vi "DIALOG_Cluster Item Selection.vi"(7 "Action":T15=enum."Bundler Insert", 8 "Error In":errorcluster, 9 "User VI Ref":refnum<vi>, 10 "Affected Items":T13, 11 "Display Items":T14[](array[typedef])) -> (0 "Error Out":errorcluster, 2 "Action Choice Out":enum32{"Choice 1", "Choice 2"}(radio), 3 "Selected Items (tags)":string[](array[string]))   [LabVIEW 2023]
doc: "Dialog to select items from the input cluster ref. \n\nFilter narrows list of items.\nDown key puts focus on tree and selects first item.\nUp and Down keps navigate tree.\nMultiple items can be selected.\n\nIn case of action \"Delete\" (\"Remove elements(s)...\" selected), list will show all elements currently displayed, else it will show all elements availabel to undle or unbundle.\n\nOutput is a list of the selected item tags.\n\nSelected element is the item clicked in a bundler node, displayed ot help user remember where an insert will happen."
uses:
  controls/action enum.ctl
  cluster/Cluster Element Description.ctl
  top/BundleMagic.ctl
  eero compliance/eero-Compliance-5m-Chamber/Code/Config/Equipment/Motion Control Max Speed.ctl
  eero compliance/eero-Compliance-5m-Chamber/Code/Scan/Spurious Emissions/controls/RSE_SA Settings Cluster.ctl
  eero compliance/eero-Compliance-5m-Chamber/Code/Equipment/rhode_schwartz/Controls/Trace Types Enum.ctl
  eero compliance/eero-Compliance-5m-Chamber/Code/Sequence/Controls/Prescan Steps Cluster.ctl
  eero compliance/eero-Compliance-5m-Chamber/Code/Controls/Start Stop Step Cluster.ctl
  eero compliance/eero-Compliance-5m-Chamber/Code/Sequence/Controls/Polarization Radio Buttons.ctl
  eero compliance/eero-Compliance-5m-Chamber/Code/Sequence/Controls/Sequence Motion Control Order Enum.ctl
  eero compliance/eero-Compliance-5m-Chamber/Code/Sequence/Controls/RSE_EUT Settings.ctl
  eero compliance/eero-Compliance-5m-Chamber/Code/Equipment/eero device driver/controls/eero model.ctl
  eero compliance/eero-Compliance-5m-Chamber/Code/Sequence/Controls/EUT Command Cluster.ctl
  eero compliance/eero-Compliance-5m-Chamber/Code/Sequence/Controls/Zoom Scan Steps Cluster.ctl
  LabVIEW-common/Controls/Get-Set Enum.ctl
panel:
  in  "Filter":string
  in  "Tree":string[](tree)
  in  "Select Unwired":bool
  out "Selected Element String":string
  in  "Action Choice Radio Buttons":enum32{"Choice 1", "Choice 2"}(radio)
  in  "Done":bool
  in  "Cluster":T12={"Cont?"=TRUE, "Config File Path"=path "", "Max Speeds"={"Mast V (cm/s)"=0.0, "Mast A (cm/s^2)"=0.0, "Turntable V (deg/s)"=0.0, "Turntable A (deg/s^2)"=0.0, "Polarization (s)"=0.0}, "Scan Speeds"={"Mast V (cm/s)"=0.0, "Mast A (cm/s^2)"=0.0, "Turntable V (deg/s)"=0.0, "Turntable A (deg/s^2)"=0.0, "Polarization (s)"=0.0}, "Sequence Order Override"=TRUE, "Sequence Timing Listbox Ref"=refnum, "Spectrum Analyzer Config"={"Start Frequency"=3000000000.0, "Stop Frequency"=18000000000.0, "Resolution BW"=1000000.0, "Video BW"=3000000.0, "Sweep Time"=1.0, "Trace 1 Detector"=1, "Trace 2 Detector"=3, "Sweep Points"=10001}, "Limit Line Enums"=[], "Calib Listbox Ref"=refnum, "Correction Paths"=[], "Seq Path"=path "", "Motion Settings"={"Mast"={"Start"=0.0, "Stop"=0.0, "Step"=0.0}, "Turntable"={"Start"=0.0, "Stop"=0.0, "Step"=0.0}, "Polarizations"={"H"=TRUE, "V"=TRUE}, "Sequence Order"=enum."Height-Pol-Angle"}, "EUT Settings"={"Model"=enum."Unico", "Command Array"=[]}, "Limit Paths"=[], "Zoom Steps"={"Mast Adjustment Range (cm)"=5.0, "Mast Step Size (cm)"=10.0, "Turntable Adjustment Range (deg)"=0.0, "Turntable Step Size (deg)"=5.0}} {"Spectrum Analyzer Config"."Trace 2 Detector" items=["", "Average", "Maximum Peak", "Minimum Peak", "RMS", "QPeak", "Cispr RMS", "Cispr Average"]; "Spectrum Analyzer Config"."Trace 1 Detector" items=["", "Average", "Maximum Peak", "Minimum Peak", "RMS", "QPeak", "Cispr RMS", "Cispr Average"]; "Spectrum Analyzer Config"."Sweep Time" format="%#_13g"; "Spectrum Analyzer Config"."Video BW" format="%#_13e"; "Spectrum Analyzer Config"."Resolution BW" format="%#_13e"; "Spectrum Analyzer Config"."Stop Frequency" format="%^.3e"; "Spectrum Analyzer Config"."Start Frequency" format="%^.3e"}
  in  "Show radio":bool
  in  "C1":T16
  # "All panes scroll to origin at runtime, so we don't have to worry about pane placements\n\nThis pane contracts at runtime and vertical splitter to left sticks to right at runtime so resizing functions happen as expected."
  # "Debug"
  # "Debug Cluster"
  # "(Use for debug if display items empty)"
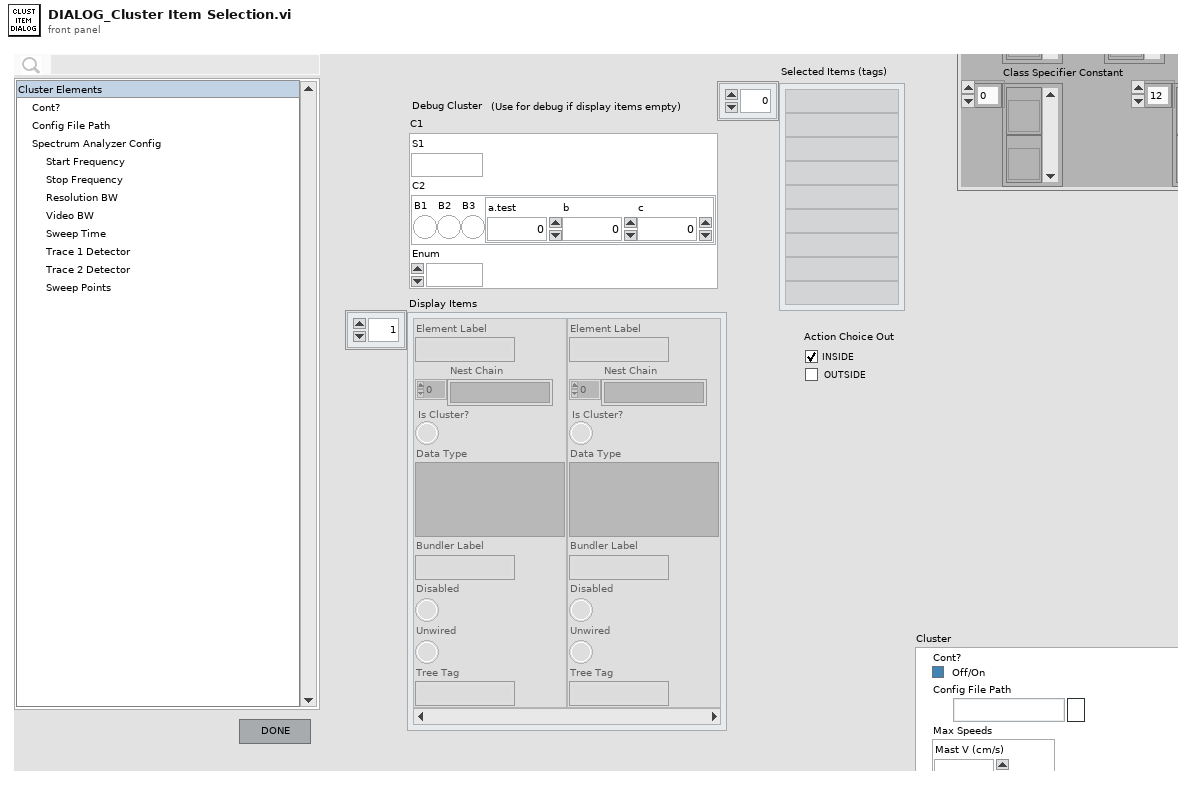
[diagram p1: front panel]
types:
  T1 = typedef "Motion Control Max Speed.ctl" = cluster{"Mast V (cm/s)":dbl, "Mast A (cm/s^2)":dbl, "Turntable V (deg/s)":dbl, "Turntable A (deg/s^2)":dbl, "Polarization (s)":dbl}
  T2 = typedef "RSE_SA Settings Cluster.ctl" = cluster{"Start Frequency":dbl, "Stop Frequency":dbl, "Resolution BW":dbl, "Video BW":dbl, "Sweep Time":dbl, "Trace 1 Detector":T3, "Trace 2 Detector":T3, "Sweep Points":u16}
  T3 = typedef "Trace Types Enum.ctl" = i32
  T4 = typedef "Prescan Steps Cluster.ctl" = cluster{"Mast":T5, "Turntable":T5, "Polarizations":T6, "Sequence Order":T7}
  T5 = typedef "Start Stop Step Cluster.ctl" = cluster{"Start":dbl, "Stop":dbl, "Step":dbl}
  T6 = typedef "Polarization Radio Buttons.ctl" = cluster{"H":bool, "V":bool}
  T7 = typedef "Sequence Motion Control Order Enum.ctl" = enum16{"Pol-Height-Angle", "Pol-Angle-Height", "Height-Angle-Pol", "Height-Pol-Angle", "Angle-Height-Pol", "Angle-Pol-Height"}
  T8 = typedef "RSE_EUT Settings.ctl" = cluster{"Model":T9, "Command Array":T10[]}
  T9 = typedef "eero model.ctl" = enum16{"Unico", "Piccino", "Cento", "Andytown-g", "Andytown-l", "Eden", "Firefly", "Trieste", "Jupiter", "Crane", "Ladro", "Merci", "Snowbird\n"}
  T10 = typedef "EUT Command Cluster.ctl" = cluster{"Command(s)":string, "Scan ID":string}
  T11 = typedef "Zoom Scan Steps Cluster.ctl" = cluster{"Mast Adjustment Range (cm)":dbl, "Mast Step Size (cm)":dbl, "Turntable Adjustment Range (deg)":dbl, "Turntable Step Size (deg)":dbl}
  T12 = cluster{"Cont?":bool, "Config File Path":path, "Max Speeds":T1, "Scan Speeds":T1, "Sequence Order Override":bool, "Sequence Timing Listbox Ref":refnum<vi>, "Spectrum Analyzer Config":T2, "Limit Line Enums":refnum<vi>[], "Calib Listbox Ref":refnum<vi>, "Correction Paths":path[], "Seq Path":path, "Motion Settings":T4, "EUT Settings":T8, "Limit Paths":path[], "Zoom Steps":T11}
  T13 = typedef "BundleMagic.ctl" = cluster{"Terminals":refnum<vi>[], "Wires":refnum<vi>[], "Named Bundler":refnum<vi>[], "Named Unbundler":refnum<vi>[], "In Place Cluster Node":refnum<vi>[], "Class Specifier Constant":refnum<vi>[], "Property Node":refnum<vi>[], "Invoke Node":refnum<vi>[], "Refnum Control":refnum<vi>[]}
  T14 = typedef "Cluster Element Description.ctl" = cluster{"Element Label":string, "Nest Chain":string[], "Is Cluster?":bool, "Data Type":variant, "Bundler Label":string, "Disabled":bool, "Unwired":bool, "Tree Tag":string}
  T15 = typedef "action enum.ctl" = enum16{"[NONE]", "Wire Bundle", "Wire Unbundle", "Terminal Unbundle", "Terminal Bundle", "Bundler Move Up", "Bundler Move Down", "Bundler Insert", "Bundler Remove", "Bundler Remove Unwired", "Bundler Rearrange", "In Place Insert", "In Place Remove", "In Place Remove Unwired", "In Place Rearrange", "Wire Properties", "Wire Method", "Terminal Properties", "Terminal Method", "Property Move Up", "Property Move Down", "Properties Insert", "Properties Remove", "Properties Remove Unwired", "Properties Rearrange", "Method Change", "Class for Constant", "Class For Control", "Class For Node", "Class Name to Clipboard"}
  T16 = cluster{"S1":string, "C2":cluster{"B1":bool, "B2":bool, "B3":bool, cluster{"a.test":dbl, "b":i32, "c":u8}}, "Enum":enum16{""}}
  T17 = typedef "Get-Set Enum.ctl" = enum16{"Get", "Set"}
  T18 = typedef "eventvkey.ctl" = enum16{"ASCII", "Enter", "Return", "Shift", "Ctrl", "Alt", "Cmd", "Opt", "Caps", "NumLock", "Clear", "Break", "Up", "Down", "Left", "Right", "Insert", "Delete", "Home", "End", "PageUp", "PageDown", "Escape", "Help", "Pause", "ScrollLock", "F1", "F2", "F3", "F4", "F5", "F6", "F7", "F8", "F9", "F10", "F11", "F12", "F13", "F14", "F15", "F16", "F17", "F18", "F19", "F20", "F21", "F22", "F23", "F24", "Play", "VolumeUp", "VolumeDown", "Mute", "Two Byte Char"}
  T19 = typedef "LVPoint32TypeDef.ctl" = cluster{"Horizontal":i32, "Vertical":i32}
  T20 = cluster{"Shift":bool, "Ctrl":bool, "Alt":bool, "Cmd":bool, "Opt":bool}
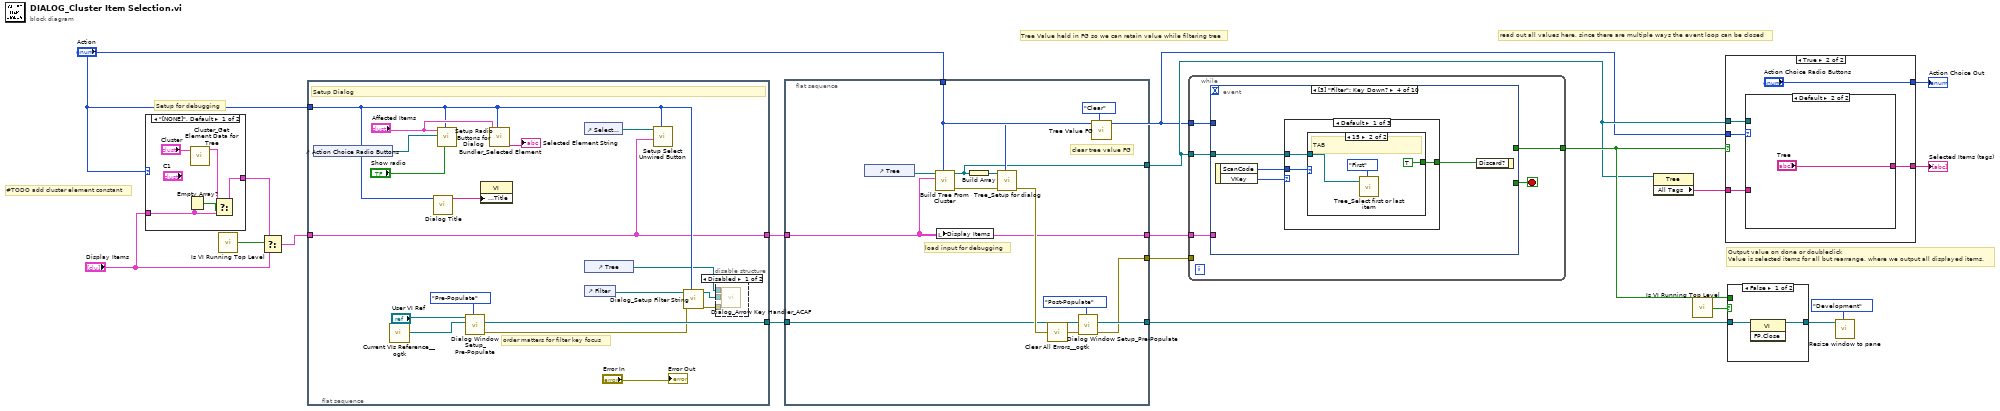
[diagram p0: block diagram]
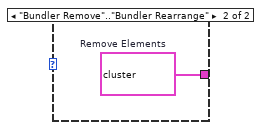
[diagram p2: hidden frame]
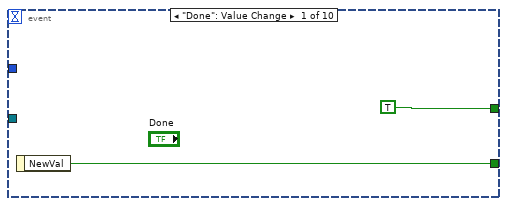
[diagram p4: hidden frame]
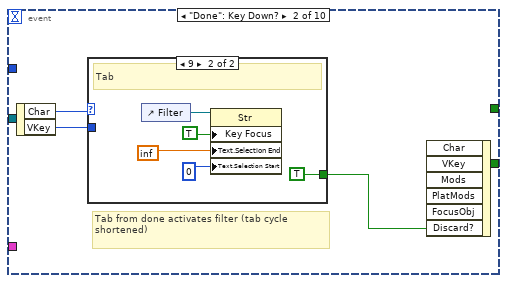
[diagram p5: hidden frame]
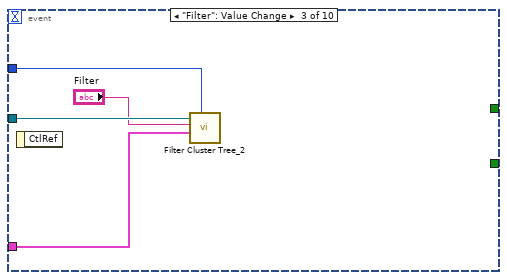
[diagram p7: hidden frame]
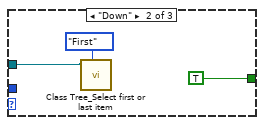
[diagram p9: hidden frame]
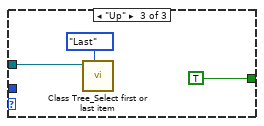
[diagram p10: hidden frame]
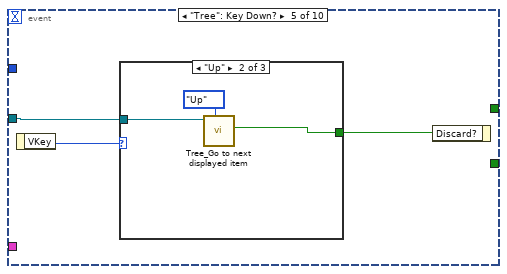
[diagram p11: hidden frame]
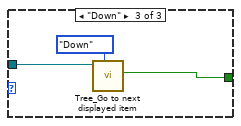
[diagram p13: hidden frame]
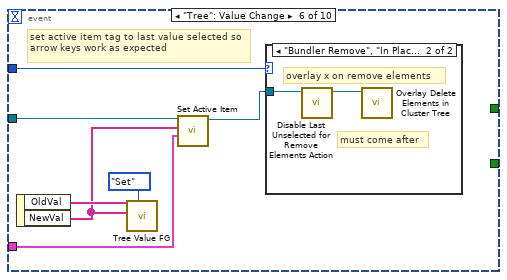
[diagram p14: hidden frame]
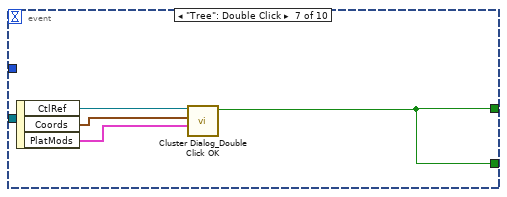
[diagram p16: hidden frame]
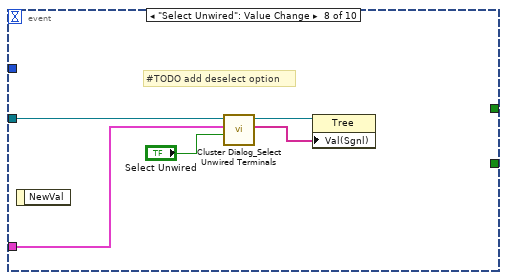
[diagram p17: hidden frame]
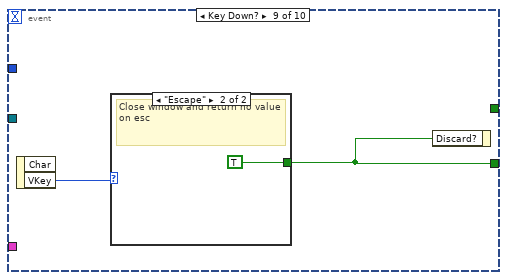
[diagram p18: hidden frame]
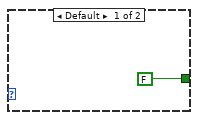
[diagram p19: hidden frame]
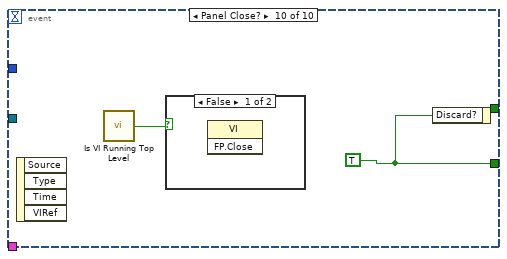
[diagram p20: hidden frame]
diagram:
  # "#TODO add cluster element constant"
  # "Setup for debugging"
  # "Tree Value held in FG so we can retain value while filtering tree"
  # "read out all values here, since there are multiple ways the event loop can be closed"
  # "Output value on done or doubleclick\nValue is selected items for all but rearrange, where we output all displayed items."
  n1 = case shown="\"[NONE]\", Default" "Action" {
    tunnel: [w21 w24] -> w4
    tunnel: "Display Items" -> [w20 _]
    frame "[NONE]", Default {
      n2 = Empty Array?(array=w20) -> (empty?=w19:bool)
      n3 = call "Cluster_Get Element Data for Tree.vi"("Data Type"="Cluster") -> ("Cluster Element Data Aray"=w22:T14[])  [unwired: 10 in]
      n4 = Select(t=w22, s=w19, f=w20) -> (s? t:f=w21:T14[])
    }
    frame "Bundler Remove".."Bundler Rearrange" {
      w24 = T14[] [{"Element Label"="N1", "Nest Chain"=[], "Is Cluster?"=FALSE, "Data Type"=variant(dbl 0.0), "Bundler Label"="N1", "Disabled"=FALSE, "Unwired"=FALSE, "Tree Tag"="0[$`~g;}N1"}, {"Element Label"="N2", "Nest Chain"=["C1"], "Is Cluster?"=TRUE, "Data Type"=variant(dbl 0.0), "Bundler Label"="C1.N2", "Disabled"=FALSE, "Unwired"=FALSE, "Tree Tag"="C1[$`~g;}C1[$`~g;}N2"}, {"Element Label"="Boolean", "Nest Chain"=["C1"], "Is Cluster?"=TRUE, "Data Type"=variant(bool FALSE), "Bundler Label"="C1.Boolean", "Disabled"=FALSE, "Unwired"=TRUE, "Tree Tag"="C2[$`~g;}C1[$`~g;}Boolean"}, {"Element Label"="C1", "Nest Chain"=[], "Is Cluster?"=FALSE, "Data Type"=variant(cluster{"N2":dbl, "Boolean":bool} {"N2"=0.0, "Boolean"=FALSE}), "Bundler Label"="C1", "Disabled"=FALSE, "Unwired"=FALSE, "Tree Tag"="3[$`~g;}C1"}, {"Element Label"="String", "Nest Chain"=[], "Is Cluster?"=FALSE, "Data Type"=variant(string ""), "Bundler Label"="String", "Disabled"=FALSE, "Unwired"=FALSE, "Tree Tag"="4[$`~g;}String"}]  # Remove Elements
    }
  }
  n5 = call "Is VI Running Top Level.vi"() -> ("Top Level?"=w5:bool)  [unwired: 5 in]
  n6 = Select(t=w4, s=w5, f="Display Items") -> (s? t:f=w3:T14[])
  n7 = flat-sequence {
    tunnel: "Action" -> [w36]
    tunnel: [w25] -> w9
    tunnel: [w32] -> w11
    tunnel: w3 -> [w25]
    frame #0 {
      # "order matters for filter key focus"
      # "Setup Dialog"
      n8 = control-ref of="Action Choice Radio Buttons"() -> (w41:refnum<vi>)
      n9 = call <userlib>:"Current VIs Reference__ogtk.vi"() -> ("Current VI's reference"=w35:refnum<vi>)  [unwired: 5 in]
      n10 = call "Dialog Title.vi"("Action"=w36) -> ("Window Title"=w39:string)  [unwired: 10 in]
      n11 = call "Setup Radio Buttons for Dialog.vi"("Show Radio"="Show radio", "Action"=w36, "Action Choice Ref"=w41, "Affected Items"="Affected Items") -> ()  [unwired: 8 in]
      n12 = call "Dialog Window Setup_Pre-Populate.vi"("Action"=enum16{"Pre-Populate", "Post-Populate"}."Pre-Populate", "Dialog VI Ref In [Parent]"=w35, "Scripted VI Ref"="User VI Ref") -> ("error out"=w29:errorcluster, "Dialog VI Ref Out"=w32:refnum<vi>)  [unwired: 7 in]
      n13 = property class="VI"("Front Panel.Title"=w39) -> ()  [unwired: 2 in, 2 out]
      n14 = call "Bundler_Selected Element.vi"("Action"=w36, "Affected Items"="Affected Items") -> ("Display String"=→"Selected Element String":string)  [unwired: 4 in, 5 out]
      n15 = control-ref of="Tree"() -> (w27:refnum<vi>)
      n16 = control-ref of="Select Unwired"() -> (w40:refnum<vi>)
      n17 = control-ref of="Filter"() -> (w30:refnum<vi>)
      n18 = call "Setup Select Unwired Button.vi"("Action"=w36, "Display Items"=w25, "Boolean in"=w40) -> ()  [unwired: 9 in]
      n19 = call "Dialog_Setup Filter String.vi"("Action"=w36, "error in"=w29, "Filter String Ref"=w30) -> ("error out"=w28:errorcluster, "Filter String Ref Out"=w26:refnum<vi>)  [unwired: 7 in]
      n20 = disable-structure shown="Disabled" {
        disable-tunnel: w28 -> [w45 _]
        disable-tunnel: w27 -> [w44 _]
        disable-tunnel: w26 -> [w43 _]
        frame Disabled {
          n21 = call "Dialog_Arrow Key Handler_ACAF.vi"("error in (no error)"=w45, "String Ref"=w43, "Tree Ref"=w44) -> ()  [unwired: 8 in, 1 out]
        }
        frame Enabled {
        }
      }
      "Error Out" <- "Error In"
    }
  }
  n22 = flat-sequence {
    tunnel: "Action" -> [w56]
    tunnel: w11 -> [w53]
    tunnel: [w52] -> w10
    tunnel: w9 -> [w46]
    tunnel: [w49] -> w8
    tunnel: [w46] -> w7
    tunnel: [w48] -> w6
    frame #0 {
      # "clear tree value FG"
      # "load input for debugging"
      n23 = control-ref of="Tree"() -> (w57:refnum<vi>)
      n24 = call "Build Tree From Cluster.vi"("Action"=w56, "Display Items"=w46, "Tree Ref"=w57) -> ("error out"=w58:errorcluster, "Tree Ref Out"=w48:refnum<vi>)  [unwired: 7 in]
      n25 = local write "Display Items"(w46) -> ()
      n26 = Build Array(w48) -> (w55:refnum<vi>[])
      n27 = call "Tree_Setup for dialog.vi"("Action"=w56, "error in"=w58, "Tree Ref"=w55) -> ("error out"=w54:errorcluster)  [unwired: 7 in, 1 out]
      n28 = call <userlib>:"Clear All Errors__ogtk.vi"("Error In"=w54) -> ("Error Out"=w50:errorcluster)  [unwired: 3 in]
      n29 = call "Dialog Window Setup_Pre-Populate.vi"("Action"=enum16{"Pre-Populate", "Post-Populate"}."Post-Populate", "error in"=w50, "Dialog VI Ref In [Parent]"=w53) -> ("error out"=w49:errorcluster, "Dialog VI Ref Out"=w52:refnum<vi>)  [unwired: 7 in]
      n30 = call "Tree Value FG.vi"("Get Set Enum"=enum16{"Get", "Set", "Clear"}."Clear") -> ()  [unwired: 10 in, 1 out]
    }
  }
  n31 = while {
    tunnel: w6 -> [w62]
    tunnel: [w61] -> w13
    tunnel: "Action" -> [w60]
    tunnel: w7 -> [w59]
    tunnel: w8 -> [_]
    stop <- w63 stop-if-true
    n32 = event shown="[3] \"Filter\": Key Down?" {
      selector: _ -> [_ _ _ _ _ _ _ _ _ _]
      dyn-events: _ -> [_ _ _ _ _ _ _ _ _ _]
      timeout: _ -> [_ _ _ _ _ _ _ _ _ _]
      tunnel: [w65 _ _ _ _ _ w115 _ w121 w126] -> w63
      tunnel: w62 -> [_ _ w77 w81 w94 w107 _ w119 _ _]
      tunnel: [TRUE _ _ _ _ _ w115 _ _ _] -> w61
      tunnel: w60 -> [_ _ w74 _ _ w109 _ _ _ _]
      tunnel: w59 -> [_ _ w75 _ _ w103 _ w120 _ _]
      event "Done": Value Change {
        n33 = event-data() -> ("NewVal"=w65:bool)  [unwired: 1 in]
      }
      event "Done": Key Down? {
        # "Tab from done activates filter (tab cycle shortened)"
        n34 = event-data() -> ("Char"=w68:i16, "VKey"=w66:T18)  [unwired: 1 in]
        n35 = case shown="9" w68 {
          tunnel: [_ TRUE ("Discard?")] -> w67
          tunnel: w66 -> [_ _]
          frame 0, Default {
          }
          frame 9 {
            # "Tab"
            n36 = control-ref of="Filter"() -> (w72:refnum<vi>)
            n37 = property class="Str"(reference=w72, "Key Focus"=TRUE, "Text.Selection End"=inf, "Text.Selection Start"=u32 0 ("Text.Selection:Start")) -> ()  [unwired: 1 in, 2 out]
          }
        }
        n38 = event-data("Discard?"=w67) -> ()  [unwired: 6 in, 1 out]
      }
      event "Filter": Value Change {
        n39 = event-data() -> ()  [unwired: 1 in, 1 out]
        n40 = call "Filter Cluster Tree_2.vi"("Action"=w74, "Display Items"=w75, "Filter Str"="Filter", "Tree Ref"=w77) -> ()  [unwired: 7 in, 1 out]
      }
      event "Filter": Key Down? {
        n41 = event-data() -> ("ScanCode"=w79:i16, "VKey"=w80:T18)  [unwired: 1 in]
        n42 = case shown="Default" w80 {
          tunnel: [w83 TRUE TRUE] -> w78
          tunnel: w81 -> [w84 w88 w92]
          tunnel: w79 -> [w82 _ _]
          frame Default {
            n43 = case shown="15" w82 {
              tunnel: w84 -> [_ w86]
              tunnel: [_ TRUE] -> w83
              frame 0, Default {
              }
              frame 15 {
                # "TAB"
                n44 = call "Tree_Select first or last item.vi"("Select Item"=enum16{"First", "Last"}."First", "Tree Ref"=w86) -> ()  [unwired: 8 in, 2 out]
              }
            }
          }
          frame "Down" {
            n45 = call "Class Tree_Select first or last item.vi"("Select Item"=enum16{"First", "Last"}."First", "Tree Ref"=w88) -> ()  [unwired: 9 in, 1 out]
          }
          frame "Up" {
            n46 = call "Class Tree_Select first or last item.vi"("Select Item"=enum16{"First", "Last"}."Last", "Tree Ref"=w92) -> ()  [unwired: 9 in, 1 out]
          }
        }
        n47 = event-data("Discard?"=w78) -> ()  [unwired: 1 in, 1 out]
      }
      event "Tree": Key Down? {
        n48 = event-data() -> ("VKey"=w96:T18)  [unwired: 1 in]
        n49 = case shown="\"Up\"" w96 {
          tunnel: [_ w97 w100] -> w95
          tunnel: w94 -> [_ w98 w101]
          frame Default {
          }
          frame "Up" {
            n50 = call "Tree_Go to next displayed item.vi"("Direction"=enum16{"Down", "Up"}."Up", "Tree ref"=w98) -> ("discard"=w97:bool)  [unwired: 7 in, 2 out]
          }
          frame "Down" {
            n51 = call "Tree_Go to next displayed item.vi"("Direction"=enum16{"Down", "Up"}."Down", "Tree ref"=w101) -> ("discard"=w100:bool)  [unwired: 7 in, 2 out]
          }
        }
        n52 = event-data("Discard?"=w95) -> ()  [unwired: 1 in, 1 out]
      }
      event "Tree": Value Change {
        # "set active item tag to last value selected so arrow keys work as expected"
        n53 = event-data() -> ("OldVal"=w106:string[], "NewVal"=w104:string[])  [unwired: 1 in]
        n54 = call "Tree Value FG.vi"("Get Set Enum"=Get-Set_Enum."Set", "NewVal"=w104, "Old Val"=w106) -> ()  [unwired: 8 in, 1 out]
        n55 = call "Set Active Item.vi"("Display Items"=w103, "NewVal"=w104, "TreeControl in"=w107) -> ("TreeControl out"=w108:refnum<vi>)  [unwired: 8 in]
        n56 = case shown="\"Bundler Remove\", \"In Place Remove\"" w109 {
          tunnel: w108 -> [_ w111]
          frame "[NONE]", Default {
          }
          frame "Bundler Remove", "In Place Remove" {
            # "overlay x on remove elements"
            # "must come after"
            n57 = call "Disable Last Unselected for Remove Elements Action.vi"("Tree Ref"=w111) -> ("Tree Ref Out"=w110:refnum<vi>)  [unwired: 8 in, 2 out]
            n58 = call "Overlay Delete Elements in Cluster Tree.vi"("Tree Ref"=w110) -> ()  [unwired: 10 in, 1 out]
          }
        }
      }
      event "Tree": Double Click {
        # "Double click to select and end entry"
        n59 = event-data() -> ("CtlRef"=w114:refnum<vi>, "Coords"=w113:T19, "PlatMods"=w112:T20)  [unwired: 1 in]
        n60 = call "Cluster Dialog_Double Click OK.vi"("PlatMods"=w112, "Coords"=w113, "TreeControl in"=w114) -> ("Valid Item Double Clicked"=w115:bool)  [unwired: 8 in]
      }
      event "Select Unwired": Value Change {
        # "#TODO add deselect option"
        n61 = event-data() -> ()  [unwired: 1 in, 1 out]
        n62 = call "Cluster Dialog_Select Unwired Terminals.vi"("Select Unwired"="Select Unwired", "Display Items"=w120, "Tree Ref"=w119) -> ("Selected items"=w116:string[], "Tree Ref Out"=w117:refnum<vi>)  [unwired: 7 in]
        n63 = property class="Tree"(reference=w117, "Val(Sgnl)"=w116) -> ()  [unwired: 1 in, 2 out]
      }
      event Key Down? {
        # "Quit on escape"
        n64 = event-data() -> ("VKey"=w122:T18)  [unwired: 1 in, 1 out]
        n65 = case shown="\"Escape\"" w122 {
          tunnel: [FALSE TRUE] -> w121
          frame Default {
          }
          frame "Escape" {
            # "Close window and return no value on esc"
          }
        }
        n66 = event-data("Discard?"=w121) -> ()  [unwired: 1 in, 1 out]
      }
      event Panel Close? {
        w126 = TRUE
        # "close and return no value on panel close"
        n67 = event-data() -> ()  [unwired: 1 in, 4 out]
        n68 = call "Is VI Running Top Level.vi"() -> ("Top Level?"=w125:bool)  [unwired: 5 in]
        n69 = case shown="False" w125 {
          frame False {
            n70 = invoke class="VI" method="FP.Close"() -> ()  [unwired: 3 in, 3 out]
          }
          frame True {
          }
        }
        n71 = event-data("Discard?"=w126) -> ()  [unwired: 1 in, 1 out]
      }
    }
  }
  n72 = property class="Tree"(reference=w6) -> ("All Tags"=w12:string[])  [unwired: 1 in, 2 out]
  n73 = call "Is VI Running Top Level.vi"() -> ("Top Level?"=w15:bool)  [unwired: 5 in]
  n74 = case shown="True" w13 {
    tunnel: [_ w131] -> w18
    tunnel: "Action" -> [_ w130]
    tunnel: w6 -> [_ w129]
    tunnel: [_ "Action Choice Radio Buttons"] -> w16
    tunnel: w12 -> [_ w127]
    frame False {
    }
    frame True {
      n75 = case shown="Default" w130 {
        tunnel: [w132 "Tree"] -> w131
        tunnel: w129 -> [w137 _]
        tunnel: w127 -> [w136 _]
        frame "Bundler Rearrange", "In Place Rearrange" {
          # "if no change, output empty arr so nothing happens"
          n76 = property class="Tree"(reference=w137) -> ("All Tags"=w133:string[])  [unwired: 1 in, 2 out]
          n77 = Not Equal?(x=w133, y=w136) -> (x != y?=w135:bool)
          n78 = Select(t=w133, s=w135, f=string[] []) -> (s? t:f=w132:string[])
        }
        frame Default {
        }
      }
    }
  }
  "Selected Items (tags)" <- w18
  "Action Choice Out" <- w16
  n79 = case shown="False" w15 {
    tunnel: w10 -> [w140 w141]
    tunnel: [w139 w141] -> w14
    tunnel: w13 -> [_ _]
    frame False {
      n80 = invoke class="VI" method="FP.Close"(reference=w140) -> (reference out=w139:refnum<vi>)  [unwired: 2 in, 2 out]
    }
    frame True {
    }
  }
  n81 = call "Resize window to pane.vi"("Mode"=enum16{"Run", "Development"}."Development", "VI Ref In"=w14) -> ()  [unwired: 8 in, 2 out]
